vi "Read (Single Digital Waveform).vi"(8 "error in (no error)":errorcluster, 9 "Maximum Time (10000ms)":u32=10000, 10 "Digital Channel (14: Digital Channel D0)":u16(ring)=14 items=["Digital Channel D0"=14, "Digital Channel D1"=15, "Digital Channel D2"=16, "Digital Channel D3"=17, "Digital Channel D4"=18, "Digital Channel D5"=19, "Digital Channel D6"=20, "Digital Channel D7"=21, "Digital Channel D8"=22, "Digital Channel D9"=23, "Digital Channel D10"=24, "Digital Channel D11"=25, "Digital Channel D12"=26, "Digital Channel D13"=27, "Digital Channel D14"=28, "Digital Channel D15"=29], 11 "VISA resource name":refnum<visa-resource-name>) -> (0 "error out":errorcluster, 2 "Digital Waveform":digitalwaveform(graph), 3 "VISA resource name out":refnum<visa-resource-name>)   [LabVIEW 2017, in "Tektronix DPO MSO 2000 4000 Series.lvlib"]
doc: "Initiates an acquisition on all channels that you enabled with the <B>Configure Digital Channel</B> VI. This VI waits for the acquisition to complete and returns the waveform for the <B>Digital Channel</B> you specify. The <B>Maximum Time</B> control specifies the maximum time to wait for operation complete in milliseconds. If the oscilloscope does not complete the acquisition within the time period you specify in <B>Maximum Time</B>, this VI returns a timeout error. A timeout error can occur when the trigger level is out of the range of the waveform.\n\nUse the tkdpo4k Fetch Waveform VI to obtain the waveforms for each of the remaining enabled <B>Source Channels</B> without initiating another acquisition.\n\n<B>Note:</B> If the instrument does not support auto-compensation for probe attenuation, adjust the scaling of the waveform data accordingly. You can adjust the scaling of the waveform data either automatically by using the <B>tkdpo4k Configure Channel VI</B> or manually by multiplying the waveform data by the probe attenuation.\n\nLabVIEW versions higher than 7.1 might display the data differently."
uses:
  Tektronix DPO MSO 2000 4000 Series.lvlib
  Data_Low Level/Fetch Waveform (Digital Waveform).vi
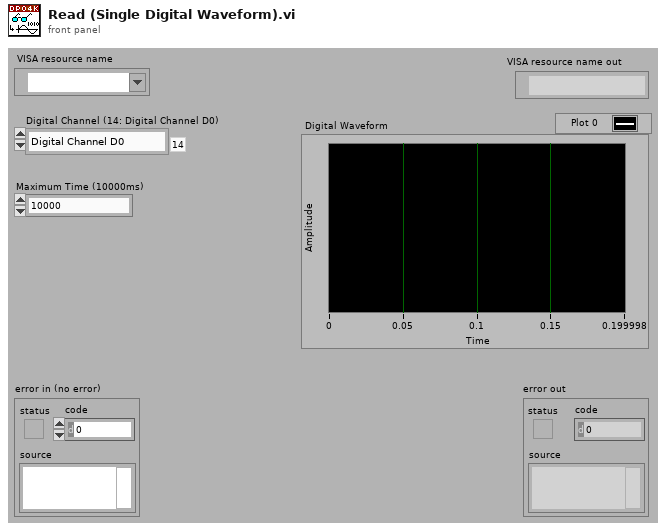
[diagram p1: front panel]
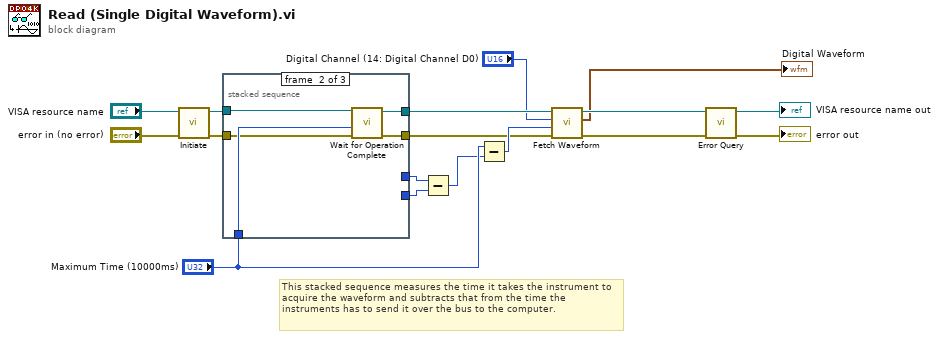
[diagram p0: block diagram]
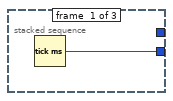
[diagram p2: hidden frame]
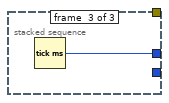
[diagram p3: hidden frame]
diagram:
  # "This stacked sequence measures the time it takes the instrument to acquire the waveform and subtracts that from the time the instruments has to send it over the bus to the computer."
  n1 = call "Initiate.vi"("error in (no error)"="error in (no error)", "VISA resource name"="VISA resource name") -> ("error out"=w12:errorcluster, "VISA resource name out"=w13:refnum<visa-resource-name>)  [unwired: 8 in]
  n2 = stacked-sequence {
    tunnel: w13 -> [_ w22 _]
    tunnel: w12 -> [_ w21 _]
    tunnel: "Maximum Time (10000ms)" -> [_ w23 _]
    tunnel: [_ w20 _] -> w7
    tunnel: [_ w19 _] -> w5
    tunnel: [_ _ w24] -> w11
    tunnel: [w18 _ _] -> w10
    frame #0 {
      n3 = Tick Count (ms)() -> (millisecond timer value=w18:u32)
    }
    frame #1 {
      n4 = call "Wait for Operation Complete.vi"("error in (no error)"=w21, "Maximum Time (10000ms)"=w23, "VISA resource name"=w22) -> ("error out"=w19:errorcluster, "VISA resource name out"=w20:refnum<visa-resource-name>)  [unwired: 7 in]
    }
    frame #2 {
      n5 = Tick Count (ms)() -> (millisecond timer value=w24:u32)
    }
  }
  n6 = Subtract(x=w11, y=w10) -> (x-y=w8:u32)
  n7 = Subtract(x="Maximum Time (10000ms)", y=w8) -> (x-y=w6:u32)
  n8 = call-poly "Fetch Waveform.vi"("error in (no error)"=w5, "Maximum Time (10000 ms)"=w6, "Digital Channel (14: Digital Channel D0)"="Digital Channel (14: Digital Channel D0)", "VISA resource name"=w7) -> ("error out"=w3:errorcluster, "Digital Waveform"=→"Digital Waveform":digitalwaveform, "VISA resource name out"=w4:refnum<visa-resource-name>)  [unwired: 5 in]
  n9 = call "Error Query.vi"("error in (no error)"=w3, "VISA resource name"=w4) -> ("error out"=→"error out":errorcluster, "VISA resource name out"=→"VISA resource name out":refnum<visa-resource-name>)  [unwired: 6 in, 2 out]
